vi "Ideal Result.vi"(8 "Error in":errorcluster, 11 "ADC in":refnum<class "ADC.lvclass">) -> (0 "Error out":errorcluster, 3 "ADC out":refnum<class "ADC.lvclass">)   [LabVIEW 2020, in "ADC.lvclass"]
uses:
  ADC.lvclass
  D:/SDLC/Class/Device/Parent/Device.lvclass
  ADC.lvclass/ADC.ctl
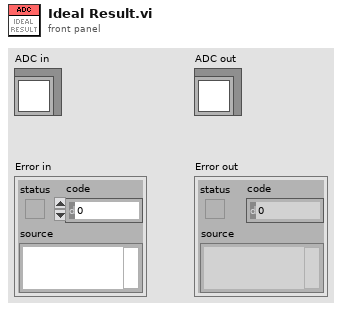
[diagram p1: front panel]
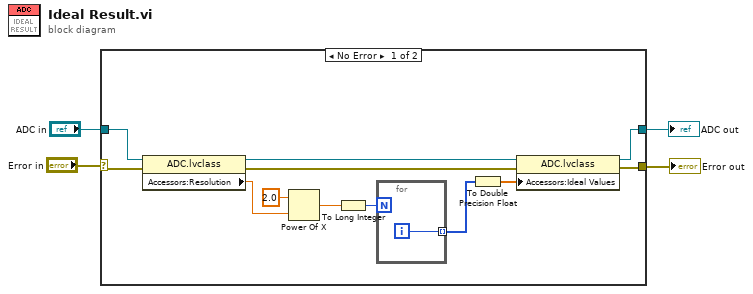
[diagram p0: block diagram]
diagram:
  n1 = case shown="No Error" "Error in" {
    selector: "Error in" -> [w15 w18]
    tunnel: "ADC in" -> [w16 w19]
    tunnel: [w6 w18] -> w2
    tunnel: [w5 w19] -> w1
    frame No Error {
      n2 = property class="ADC.lvclass"(reference=w16, error in=w15) -> (reference out=w10:refnum<class "ADC.lvclass">, error out=w9:errorcluster, "Accessors:Resolution"=w13:dbl)
      n3 = Power Of X(1:w13, 2:2.0 ("y")) -> (0:w12:dbl)
      n4 = To Long Integer(number=w12) -> (32bit integer=w11:i32)
      n5 = for {
        N: w11 -> [_]
        tunnel: [w17] -> w8 mode=indexing
        i -> [w17]
      }
      n6 = To Double Precision Float(number=w8) -> (double precision float=w7:dbl[])
      n7 = property class="ADC.lvclass"(reference=w10, error in=w9, "Accessors:Ideal Values"=w7) -> (reference out=w5:refnum<class "ADC.lvclass">, error out=w6:errorcluster)
    }
    frame Error {
    }
  }
  "Error out" <- w2
  "ADC out" <- w1
